vi "Alm.vi"(8 "error in (no error)":errorcluster caption="错误输入（无错误）", 11 "AllControls Out":T1) -> ()   [LabVIEW 2017]
uses:
  Ctrls/AllControls.ctl
  ComVIS/_OpenG/comparison/comparison.llb/1D Boolean Array Changed__ogtk.vi
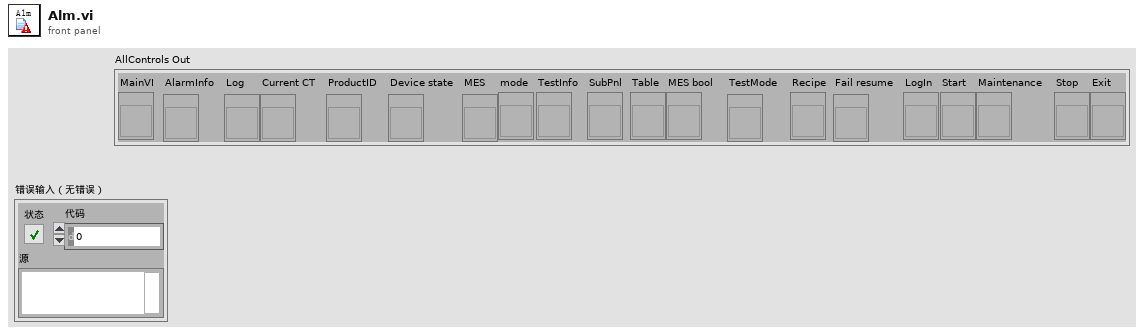
[diagram p1: front panel]
types:
  T1 = typedef "AllControls.ctl" = cluster{"MainVI":refnum<vi>, "AlarmInfo":refnum<vi>, "Log":refnum<vi>, "Current CT":refnum<vi>, "ProductID":refnum<vi>, "Device state":refnum<vi>, "MES":refnum<vi>, "mode":refnum<vi>, "TestInfo":refnum<vi>, "SubPnl":refnum<vi>, "Table":refnum<vi>, "MES bool":refnum<vi>, "TestMode":refnum<vi>, "Recipe":refnum<vi>, "Fail resume":refnum<vi>, "LogIn":refnum<vi>, "Start":refnum<vi>, "Maintenance":refnum<vi>, "Stop":refnum<vi>, "Exit":refnum<vi>}
  T2 = typedef "HD Config.ctl" = cluster{" PC":cluster{"PC Address":u8[], "PC Port":i32}, "FCO":cluster{"COM":refnum<visa-resource-name>, "Baudrate":u32}, "DC Power ":cluster{"COM":refnum<visa-resource-name>, "Baudrate":u32}, "PW3336":cluster{"COM":refnum<visa-resource-name>, "Baudrate":u32}, "Lefoo":cluster{"COM":refnum<visa-resource-name>, "Baudrate":u32}, "AI Model":cluster{"COM":refnum<visa-resource-name>, "Baudrate":u32}, "DIPC":cluster{"COM":refnum<visa-resource-name>}, "RFID":cluster{"IP Address":string, "Port":u16, "Retry":u16}, "Motor":cluster{"COM":refnum<visa-resource-name>, "Baudrate":u32}, "Fail_resume_mode":bool, "GRR":bool}
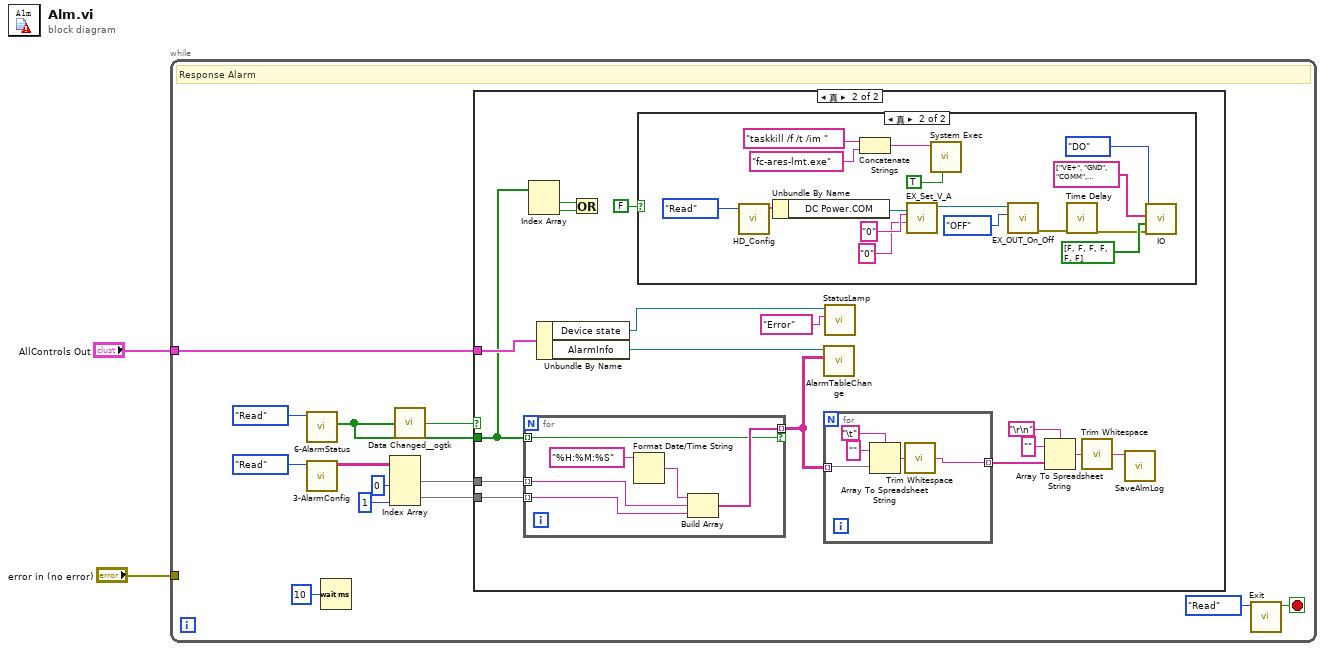
[diagram p0: block diagram]
diagram:
  n1 = while {
    tunnel: "AllControls Out" -> [w12]
    tunnel: "error in (no error)" -> [_]
    stop <- w15 stop-if-true
    # "Response Alarm"
    n2 = call "6-AlarmStatus.vi"("Step"=enum16{"Initial", "Write", "Read"}."Read") -> ("AlarmValue Out"=w3:bool[])  [unwired: 9 in, 1 out]
    n3 = call "3-AlarmConfig.vi"("Step"=enum16{"Initial", "Write", "Read"}."Read") -> ("AlarmConfig Out"=w9:string[][])  [unwired: 9 in, 1 out]
    n4 = Wait (ms)(milliseconds to wait=u32 10 ("等待时间（毫秒）")) -> ()  [unwired: 1 out]
    n5 = Index Array(array=w9, index (col) #1=0 ("禁用的索引 (列)"), index (col) #2=1 ("索引 (列)")) -> (element #1=w6:string[], element #2=w5:string[])  [unwired: 2 in]
    n6 = call-poly "Data Changed__ogtk.vi"("1D Boolean Array"=w3) -> ("Changed"=w4:bool)
    n7 = case shown="真" w4 {
      tunnel: w6 -> [_ w31]
      tunnel: w5 -> [_ w30]
      tunnel: w3 -> [_ w19]
      tunnel: w12 -> [_ w29]
      frame False {
      }
      frame True {
        n8 = for {
          tunnel: w31 -> [w56] mode=indexing
          tunnel: w30 -> [w55] mode=indexing
          tunnel: w19 -> [w53] mode=indexing
          tunnel: [w54] -> w23 mode=indexing if=w53
          n9 = Format Date/Time String(time format string (%c)="%H:%M:%S" ("时间格式字符串(%c)")) -> (date/time string=w57:string)  [unwired: 2 in]
          n10 = Build Array(w57, w56, w55) -> (w54:string[])
        }
        n11 = Index Array(array=w19) -> (element #1=w17:bool, element #2=w18:bool)  [unwired: 2 in]
        n12 = Unbundle By Name(w29) -> ("Device state"=w20:refnum<vi>, "AlarmInfo"=w24:refnum<vi>)
        n13 = Or(x=w17, y=w18) -> ()  [unwired: 1 out]
        n14 = case shown="真" FALSE {
          frame False {
          }
          frame True {
            n15 = call "HD_Config.vi"("Step"=enum16{"Initial", "Write", "Read"}."Read") -> ("HD Config out"=w45:T2)  [unwired: 9 in, 1 out]
            n16 = Unbundle By Name(w45) -> ("DC Power.COM"=w39:refnum<visa-resource-name>)
            n17 = Concatenate Strings("taskkill /f /t /im " ("字符串"), "fc-ares-lmt.exe" ("processName")) -> (w34:string)
            n18 = call "EX_Set_V_A.vi"("current"="0", "voltage"="0", "VISA resource name"=w39) -> ("VISA资源名称输出"=w38:refnum<visa-resource-name>)  [unwired: 7 in, 1 out]
            n19 = call <vilib>:"System Exec.vi"("run minimized? (F)"=TRUE, "command line"=w34) -> ()  [unwired: 6 in, 4 out]
            n20 = call "EX_OUT_On_Off.vi"("Mode"=enum16{"ON", "OFF"}."OFF", "VISA resource name"=w38) -> ("error out"=w42:errorcluster)  [unwired: 8 in, 1 out]
            n21 = call "Time Delay"("error in (no error)"=w42) -> ("error out"=w37:errorcluster)  [unwired: 10 in]
            n22 = call "IO.vi"("错误常量"=w37, "DO DATA"=bool[] [FALSE, FALSE, FALSE, FALSE, FALSE, FALSE] ("Writel_IO"), "IO Name"=string[] ["VE+", "GND", "COMM", "Sense+", "4V5", "Sense-"], "IO?"=enum16{"DI", "DO"}."DO") -> ()  [unwired: 5 in, 3 out]
          }
        }
        n23 = call "AlarmTableChange.vi"("AlarmData"=w23, "AlarmInfo"=w24) -> ()  [unwired: 9 in, 1 out]
        n24 = for {
          tunnel: w23 -> [w52] mode=indexing
          tunnel: [w48] -> w26 mode=indexing
          n25 = Array To Spreadsheet String(delimiter (Tab)="\t", array=w52, 3:"" ("format string")) -> (spreadsheet string=w49:string)
          n26 = call <vilib>:"Trim Whitespace.vi"("string"=w49) -> ("trimmed string"=w48:string)  [unwired: 1 in]
        }
        n27 = call "StatusLamp.vi"("State"="Error", "Boolean输入"=w20) -> ()  [unwired: 9 in, 1 out]
        n28 = Array To Spreadsheet String(delimiter (Tab)="\r\n", array=w26, 3:"" ("format string")) -> (spreadsheet string=w25:string)
        n29 = call <vilib>:"Trim Whitespace.vi"("string"=w25) -> ("trimmed string"=w22:string)  [unwired: 1 in]
        n30 = call "SaveAlmLog.vi"("AlmLog"=w22) -> ()  [unwired: 10 in, 1 out]
      }
    }
    n31 = call "Exit.vi"("Step"=enum16{"Initial", "Write", "Read"}."Read" ("step")) -> ("Exit Out"=w15:bool)  [unwired: 9 in, 1 out]
  }
